vi "Stack Temp HMI Screen Dev (HOA).vi"() -> ()   [LabVIEW 2023]
panel:
  out "Auto/Man":bool
  out "On/Off":bool
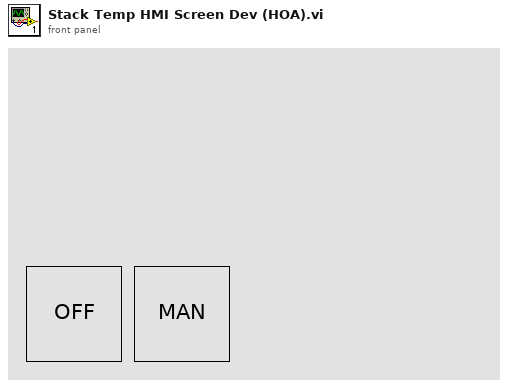
[diagram p1: front panel]
types:
  T1 = typedef "imagedata.ctl" = cluster{"image type":i32, "image depth":i32, "image":u8[], "mask":u8[], "colors":u32[], "Rectangle":cluster{"left":i16, "top":i16, "right":i16, "bottom":i16}}
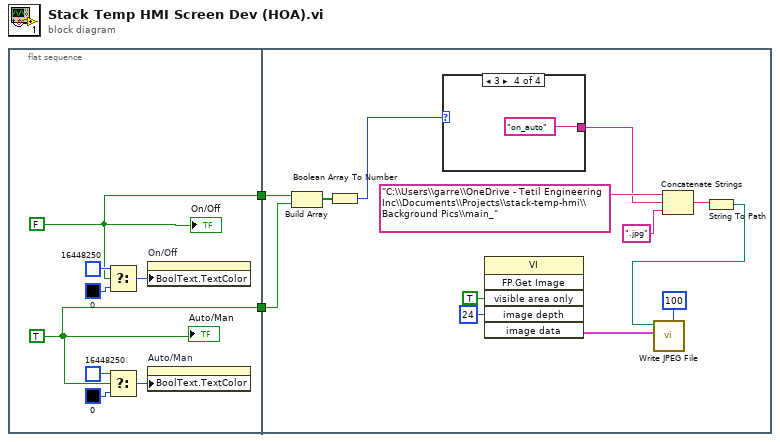
[diagram p0: block diagram]
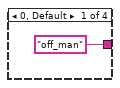
[diagram p2: hidden frame]
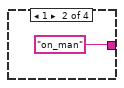
[diagram p3: hidden frame]
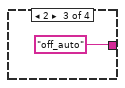
[diagram p4: hidden frame]
diagram:
  n1 = flat-sequence {
    tunnel: [w4] -> w2
    tunnel: [w3] -> w1
    tunnel: w2 -> [w15]
    tunnel: w1 -> [w14]
    frame #0 {
      w4 = TRUE ("s")
      w3 = FALSE ("s")
      n2 = Select(t=u32 16448250 ("Boolean Text.Text Colors:Text Color"), s=w3, f=u32 0 ("Boolean Text.Text Colors:Text Color")) -> (s? t:f=w8:u32)
      n3 = Select(t=u32 16448250 ("Boolean Text.Text Colors:Text Color"), s=w4, f=u32 0 ("Boolean Text.Text Colors:Text Color")) -> (s? t:f=w7:u32)
      n4 = property on="On/Off" class="Bool"("BoolText.TextColor"=w8) -> ()  [unwired: 2 in, 2 out]
      n5 = property on="Auto/Man" class="Bool"("BoolText.TextColor"=w7) -> ()  [unwired: 2 in, 2 out]
      "On/Off" <- w3
      "Auto/Man" <- w4
    }
    frame #1 {
      n6 = Build Array(w14, w15) -> (w13:bool[])
      n7 = Boolean Array To Number(Boolean array=w13) -> (number=w12:u32)
      n8 = case shown="3" w12 {
        tunnel: ["off_man" ("string") "on_man" ("string") "off_auto" ("string") "on_auto" ("string")] -> w11
        frame 0, Default {
        }
        frame 1 {
        }
        frame 2 {
        }
        frame 3 {
        }
      }
      n9 = invoke class="VI" method="FP.Get Image"("visible area only"=TRUE ("Visible Area Only"), "image depth"=24 ("Image Depth")) -> ("image data"=w22:T1)  [unwired: 4 in, 5 out]
      n10 = Concatenate Strings("C:\\Users\\garre\\OneDrive - Tetil Engineering Inc\\Documents\\Projects\\stack-temp-hmi\\Background Pics\\main_", w11, ".jpg" ("string")) -> (w17:string)
      n11 = String To Path(string=w17) -> (path=w19:path)
      n12 = call <vilib>:"Write JPEG File.vi"("quality (80)"=100, "image data"=w22, "path to JPEG file"=w19) -> ()  [unwired: 7 in, 2 out]
    }
  }
